vi "front_panel.vi"() -> ()   [LabVIEW 2019]
panel:
  out "Detected white pixels:":string
  out "Detected blue pixels:":string
  out "Detected red 2 pixels:":string
  out "Detected red pixels:":string
  out "Detected green pixels:":string
  out "Detected yellow pixels:":string
  out "Status:":bool
  out "Detected color:":string
  out "White mask:":picture
  out "Blue mask:":picture
  out "Red 2 (magenta) mask:":picture
  out "Red mask:":picture
  out "Green mask:":picture
  out "Yellow mask:":picture
  out "Current time:":string
  out "Current image:":picture
  in  "stop":bool
  in  "Next":bool
  # "PIxel count by color:"
  # "Authors: Bogdan Marinski, Konstantin Boev, Nikolai Kirilov, Raino Stefanov; Technical University of Sofia, faculty of Automatics, 2019/2020"
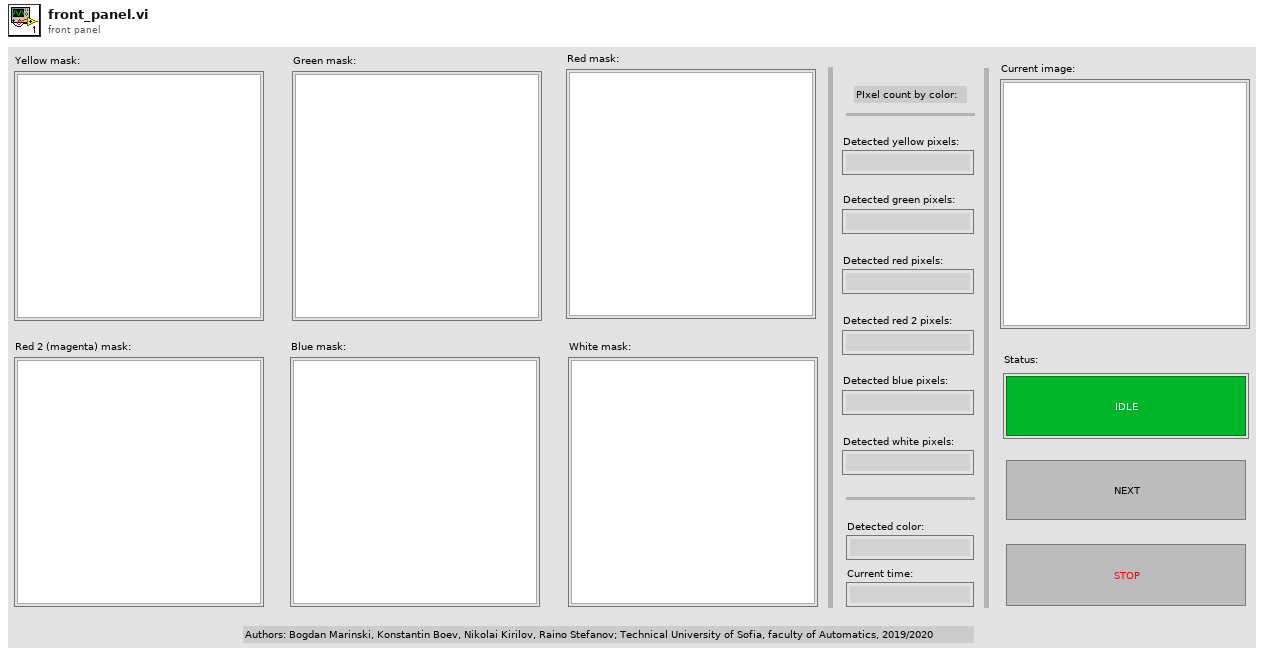
[diagram p1: front panel]
types:
  T1 = typedef "imagedata.ctl" = cluster{"image type":i32, "image depth":i32, "image":u8[], "mask":u8[], "colors":u32[], "Rectangle":cluster{"left":i16, "top":i16, "right":i16, "bottom":i16}}
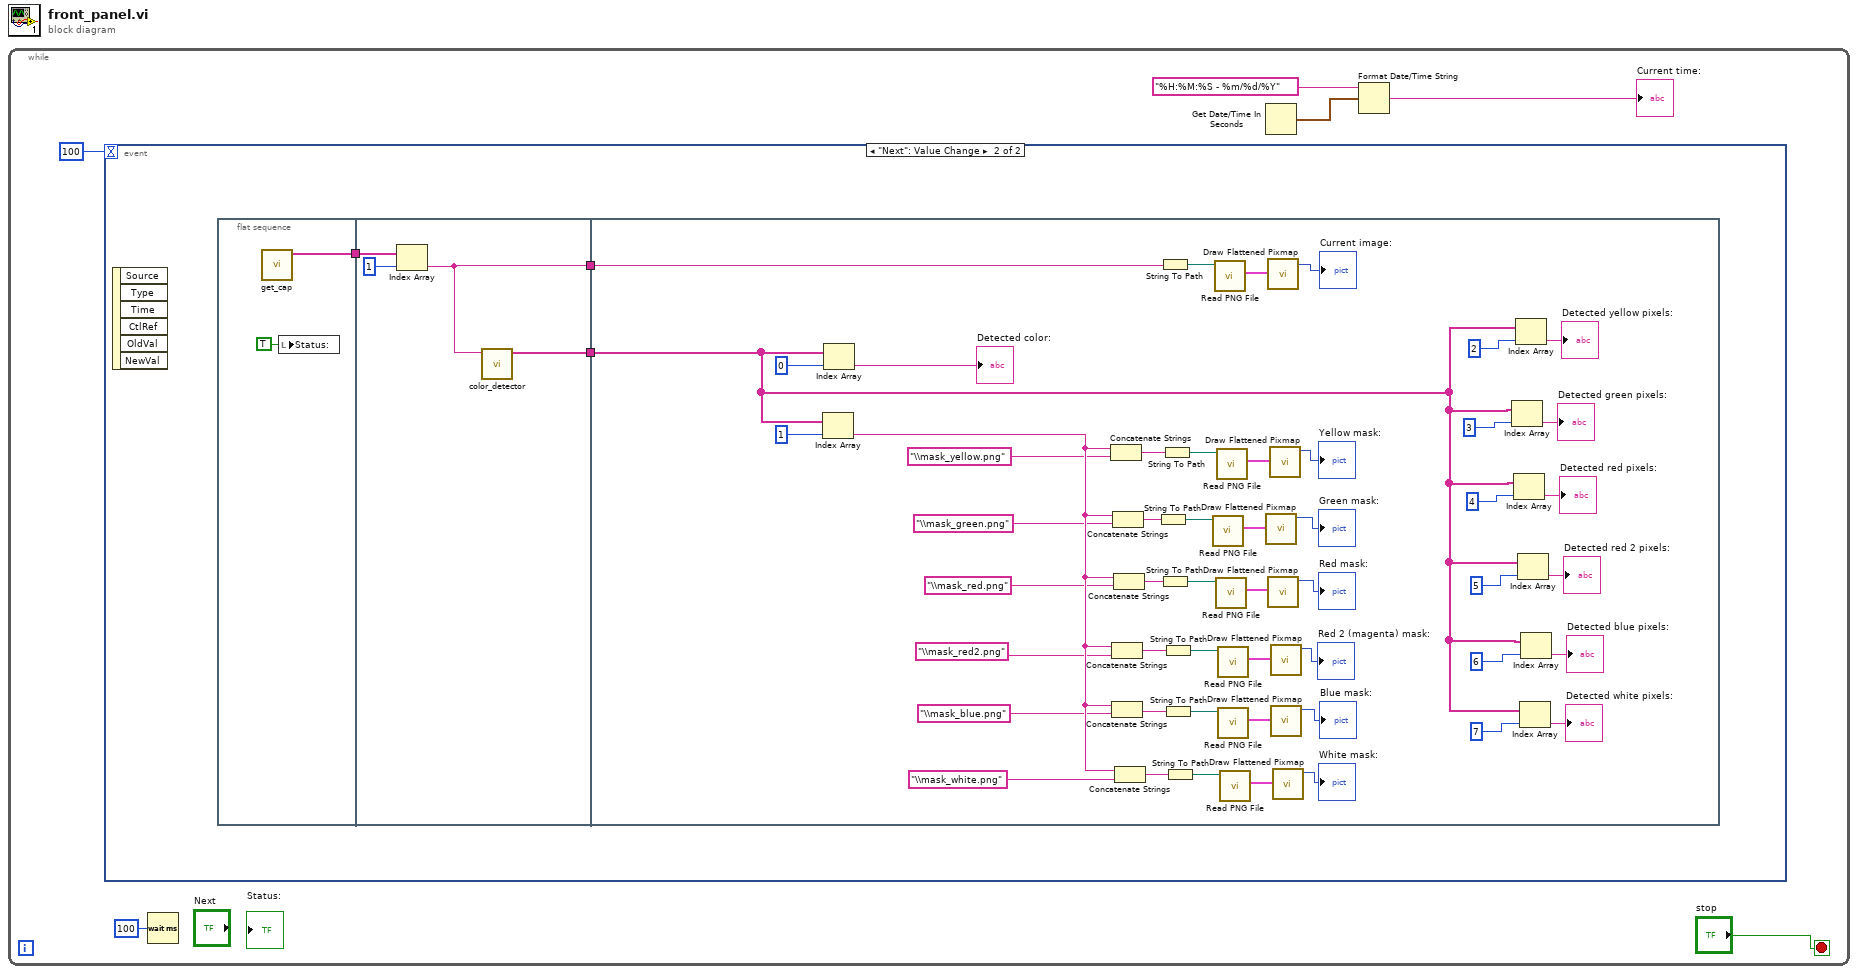
[diagram p0: block diagram]
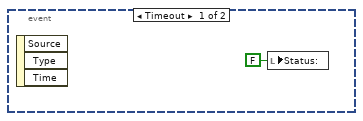
[diagram p2: hidden frame]
diagram:
  n1 = while {
    stop <- "stop" stop-if-true
    n2 = event shown="[1] \"Next\": Value Change" {
      selector: _ -> [_ _]
      dyn-events: _ -> [_ _]
      timeout: 100 -> [_ _]
      event Timeout {
        n3 = event-data() -> ()  [unwired: 1 in, 3 out]
        n4 = local write "Status:"(FALSE ("Status:")) -> ()
      }
      event "Next": Value Change {
        n5 = event-data() -> ()  [unwired: 1 in, 6 out]
        n6 = flat-sequence {
          tunnel: [w12] -> w10
          tunnel: [w13] -> w9
          tunnel: [w14] -> w8
          tunnel: w10 -> [w16]
          tunnel: w9 -> [w19]
          tunnel: w8 -> [w18]
          frame #0 {
            n7 = call "get_cap.vi"() -> ("return type"=w12:string[])  [unwired: 11 in]
            n8 = local write "Status:"(TRUE ("Status:")) -> ()
          }
          frame #1 {
            n9 = Index Array(array=w16, index=1) -> (element=w13:string)
            n10 = call "color_detector.vi"("return type in"=w13) -> ("return type out"=w14:string[])  [unwired: 10 in]
          }
          frame #2 {
            n11 = Index Array(array=w18, index=1) -> (element=w40:string)
            n12 = Index Array(array=w18, index=0) -> (element=→"Detected color:":string)
            n13 = Concatenate Strings(w40, "\\mask_yellow.png" ("string")) -> (w46:string)
            n14 = Concatenate Strings(w40, "\\mask_red2.png" ("string")) -> (w43:string)
            n15 = Concatenate Strings(w40, "\\mask_blue.png" ("string")) -> (w44:string)
            n16 = Concatenate Strings(w40, "\\mask_green.png" ("string")) -> (w41:string)
            n17 = Concatenate Strings(w40, "\\mask_red.png" ("string")) -> (w42:string)
            n18 = Concatenate Strings(w40, "\\mask_white.png" ("string")) -> (w45:string)
            n19 = String To Path(string=w41) -> (path=w61:path)
            n20 = String To Path(string=w19) -> (path=w65:path)
            n21 = String To Path(string=w42) -> (path=w59:path)
            n22 = String To Path(string=w46) -> (path=w63:path)
            n23 = String To Path(string=w43) -> (path=w57:path)
            n24 = String To Path(string=w44) -> (path=w55:path)
            n25 = String To Path(string=w45) -> (path=w53:path)
            n26 = call <vilib>:"Read PNG File.vi"("path to PNG file"=w61) -> ("image data"=w62:T1)  [unwired: 8 in, 2 out]
            n27 = call <vilib>:"Read PNG File.vi"("path to PNG file"=w65) -> ("image data"=w67:T1)  [unwired: 8 in, 2 out]
            n28 = call <vilib>:"Read PNG File.vi"("path to PNG file"=w59) -> ("image data"=w60:T1)  [unwired: 8 in, 2 out]
            n29 = call <vilib>:"Read PNG File.vi"("path to PNG file"=w63) -> ("image data"=w64:T1)  [unwired: 8 in, 2 out]
            n30 = call <vilib>:"Read PNG File.vi"("path to PNG file"=w57) -> ("image data"=w58:T1)  [unwired: 8 in, 2 out]
            n31 = call <vilib>:"Read PNG File.vi"("path to PNG file"=w55) -> ("image data"=w56:T1)  [unwired: 8 in, 2 out]
            n32 = call <vilib>:"Read PNG File.vi"("path to PNG file"=w53) -> ("image data"=w54:T1)  [unwired: 8 in, 2 out]
            n33 = call <vilib>:"Draw Flattened Pixmap.vi"("image data"=w62) -> ("new picture"=→"Green mask:":picture)  [unwired: 8 in]
            n34 = call <vilib>:"Draw Flattened Pixmap.vi"("image data"=w67) -> ("new picture"=→"Current image:":picture)  [unwired: 8 in]
            n35 = call <vilib>:"Draw Flattened Pixmap.vi"("image data"=w60) -> ("new picture"=→"Red mask:":picture)  [unwired: 8 in]
            n36 = call <vilib>:"Draw Flattened Pixmap.vi"("image data"=w64) -> ("new picture"=→"Yellow mask:":picture)  [unwired: 8 in]
            n37 = call <vilib>:"Draw Flattened Pixmap.vi"("image data"=w58) -> ("new picture"=→"Red 2 (magenta) mask:":picture)  [unwired: 8 in]
            n38 = call <vilib>:"Draw Flattened Pixmap.vi"("image data"=w56) -> ("new picture"=→"Blue mask:":picture)  [unwired: 8 in]
            n39 = call <vilib>:"Draw Flattened Pixmap.vi"("image data"=w54) -> ("new picture"=→"White mask:":picture)  [unwired: 8 in]
            n40 = Index Array(array=w18, index=3) -> (element=→"Detected green pixels:":string)
            n41 = Index Array(array=w18, index=4) -> (element=→"Detected red pixels:":string)
            n42 = Index Array(array=w18, index=2) -> (element=→"Detected yellow pixels:":string)
            n43 = Index Array(array=w18, index=5) -> (element=→"Detected red 2 pixels:":string)
            n44 = Index Array(array=w18, index=7) -> (element=→"Detected white pixels:":string)
            n45 = Index Array(array=w18, index=6) -> (element=→"Detected blue pixels:":string)
          }
        }
      }
    }
    n46 = Wait (ms)(milliseconds to wait=u32 100) -> ()  [unwired: 1 out]
    n47 = Get Date/Time In Seconds() -> (seconds since 1Jan1904=w4:timestamp)
    n48 = Format Date/Time String(time format string (%c)="%H:%M:%S - %m/%d/%Y", seconds (now)=w4) -> (date/time string=→"Current time:":string)  [unwired: 1 in]
  }
